vi "Destroy ByteArray Buffer.vi"(8 "error in":errorcluster, 9 "Return Elements (T)":bool=TRUE, 11 "Buffer":refnum<data-value>) -> (0 "error out":errorcluster, 2 "bytes":u8[](array[numeric]) format="%02x")   [LabVIEW 2013, in "ByteBuffer.lvclass"]
doc: "This VI releases resources that have been created for the ring buffer."
uses:
  ByteBuffer.lvclass
  VariantBuffer/VariantBuffer.lvclass
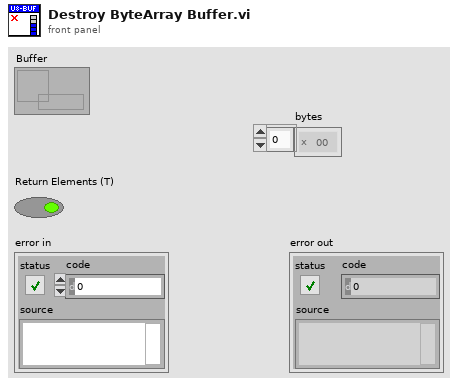
[diagram p1: front panel]
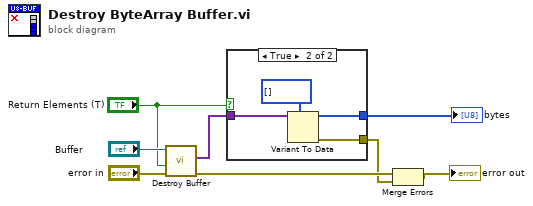
[diagram p0: block diagram]
diagram:
  n1 = call "Destroy Buffer.vi"("error in"="error in", "Return Elements (T)"="Return Elements (T)", "Buffer"="Buffer") -> ("error out"=w4:errorcluster, "elements"=w5:variant[])  [unwired: 7 in]
  n2 = case shown="True" "Return Elements (T)" {
    tunnel: [_ w10] -> w8
    tunnel: w5 -> [_ w11]
    tunnel: [_ w9] -> w3
    frame False {
    }
    frame True {
      n3 = Variant To Data(type=u8[] [] ("bytes"), Variant=w11) -> (data=w10:u8[], error out=w9:errorcluster)  [unwired: 1 in]
    }
  }
  "bytes" <- w8
  n4 = Merge Errors(w4, w3) -> (→"error out":errorcluster)
